vi "SP_GetZTheta.vi"(8 "error in (no error)":errorcluster, 11 "SemiProbe in":refnum<class "SemiProbe.lvclass">) -> (0 "error out":errorcluster, 1 "Theta out [mdeg]":dbl, 2 "Z out [µm]":dbl, 3 "SemiProbe out":refnum<class "SemiProbe.lvclass">)   [LabVIEW 2013, in "SemiProbe.lvclass"]
uses:
  SemiProbe.lvclass
  <vilib>/regexp/Match Regular Expression.xnode
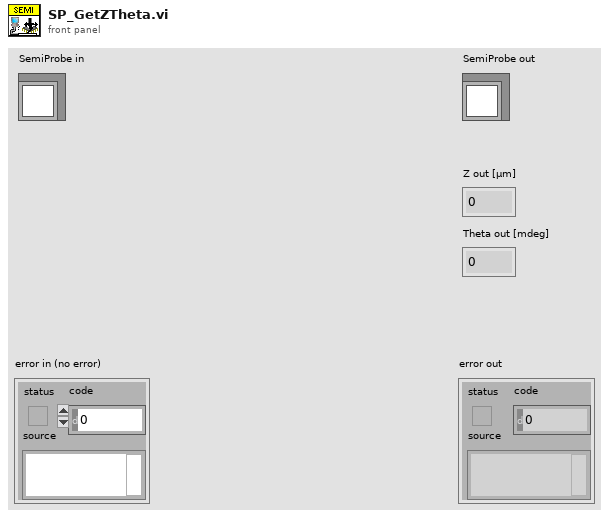
[diagram p1: front panel]
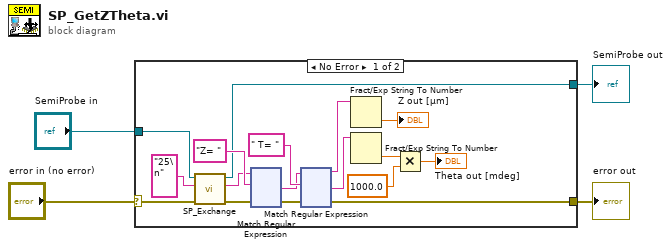
[diagram p0: block diagram]
diagram:
  n1 = case shown="No Error" "error in (no error)" {
    selector: "error in (no error)" -> [w21 w251]
    tunnel: [w11 w251] -> w3
    tunnel: [w10 w250] -> w1
    tunnel: "SemiProbe in" -> [w20 w250]
    frame No Error {
      n2 = call-dynamic "SP_Exchange.vi"("error in (no error)"=w21, "command"="25\n", "SemiProbe in"=w20) -> ("error out"=w17:errorcluster, "answer"=w13:string, "SemiProbe out"=w10:refnum<class "SemiProbe.lvclass">)  [unwired: 4 in, 2 out]
      n3 = xnode "Match Regular Expression"("input string"=w13, "regular expression"="Z= ", "error in"=w17) -> ("after match"=w15:string, "error out"=w18:errorcluster)  [unwired: 3 in, 3 out]
      n4 = xnode "Match Regular Expression"("input string"=w15, "regular expression"=" T= ", "error in"=w18) -> ("before match"=w12:string, "after match"=w9:string, "error out"=w11:errorcluster)  [unwired: 3 in, 2 out]
      n5 = Fract/Exp String To Number(string=w12) -> (number=→"Z out [µm]":dbl)  [unwired: 3 in, 1 out]
      n6 = Fract/Exp String To Number(string=w9) -> (number=w5:dbl)  [unwired: 3 in, 1 out]
      n7 = Multiply(x=w5, y=1000.0) -> (x*y=→"Theta out [mdeg]":dbl)
    }
    frame Error {
    }
  }
  "error out" <- w3
  "SemiProbe out" <- w1
